vi "P4CMD Compare Files.vi"(4 "version":string, 6 "compare options":T1, 7 "advanced options":variant, 8 "error in (no error)":errorcluster, 9 "compare method":T2 items=["source control provider default", "contents (silent)", "checksum (silent)", "time (silent)"], 10 "file path":path, 11 "source control reference in":T3) -> (0 "error out":errorcluster, 2 "status message":string, 3 "source control reference out":T3, 5 "file differs?":bool)   [LabVIEW 2020, in "NI_SCC_P4CMD.lvlib"]
uses:
  <vilib>/SourceControl/Providers/P4CMD/NI_SCC_P4CMD.lvlib
  <vilib>/SourceControl/sccapi/SCCAPI Refnum.ctl
  <vilib>/SourceControl/sccapi/SCCAPI Compare Method.ctl
  <vilib>/SourceControl/sccapi/SCCAPI Compare Options.ctl
  <vilib>/SourceControl/Providers/P4CMD/P4CMD Operations.ctl
  <vilib>/SourceControl/support/SCCSup Message Strings GLBL.vi
  <vilib>/SourceControl/sccapi/NI_SCC.lvlib
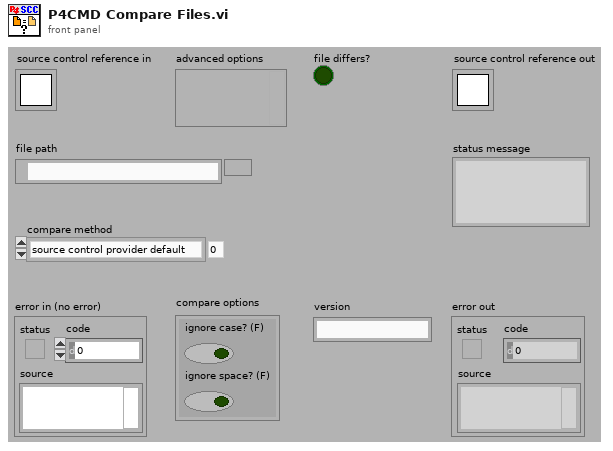
[diagram p1: front panel]
types:
  T1 = typedef "NI_SCC.lvlib/SCCAPI Compare Options.ctl" = cluster{"ignore case? (F)":bool, "ignore space? (F)":bool}
  T2 = typedef "NI_SCC.lvlib/SCCAPI Compare Method.ctl" = u16
  T3 = typedef "NI_SCC.lvlib/SCCAPI Refnum.ctl" = refnum<k1>
  T4 = typedef "NI_SCC_P4CMD.lvlib/P4CMD Operations.ctl" = enum16{"get all clients", "get all users", "describe changelist", "sync from depot", "open for edit", "submit to depot", "revert", "add to depot", "remove from depot", "print files revisions", "compare client file", "print depot file contents", "list opened files", "get file info", "lock files", "edit changelist spec", "info", "set variables"}
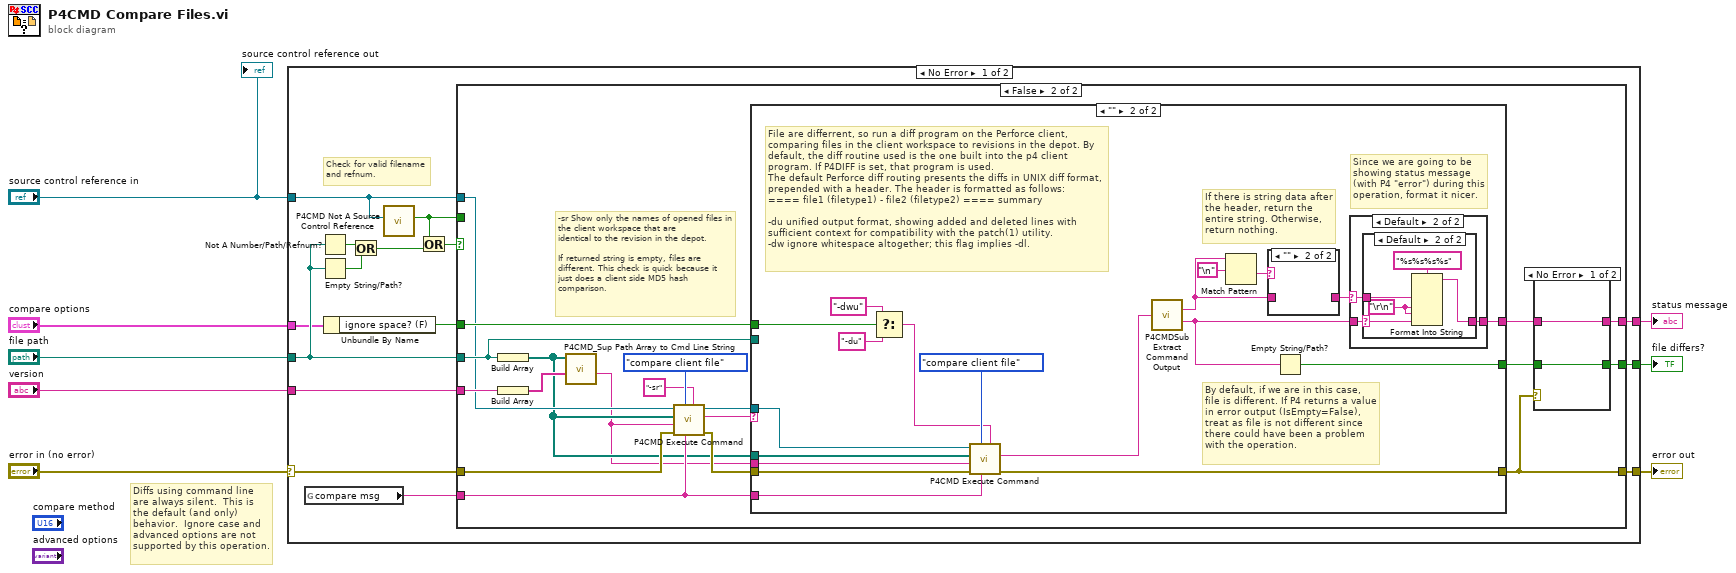
[diagram p0: block diagram]
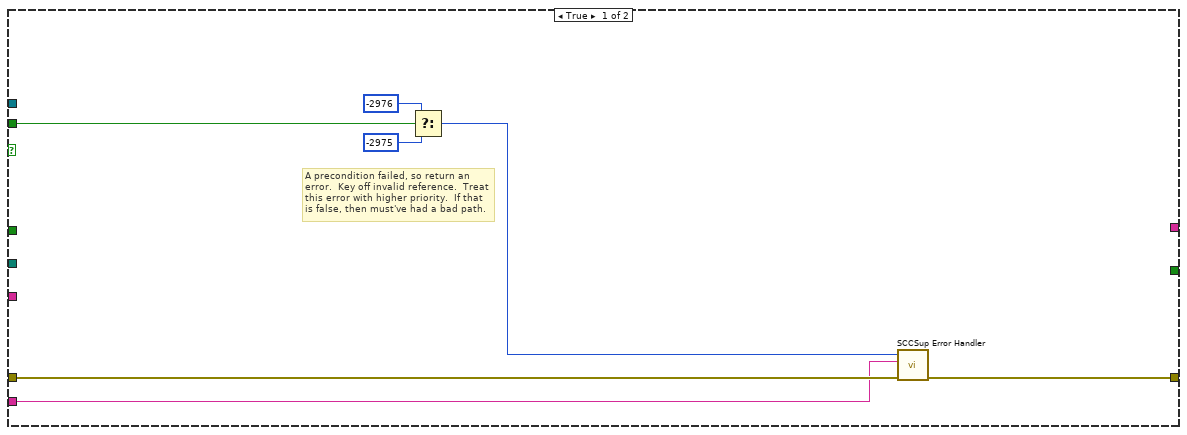
[diagram p2: hidden frame]
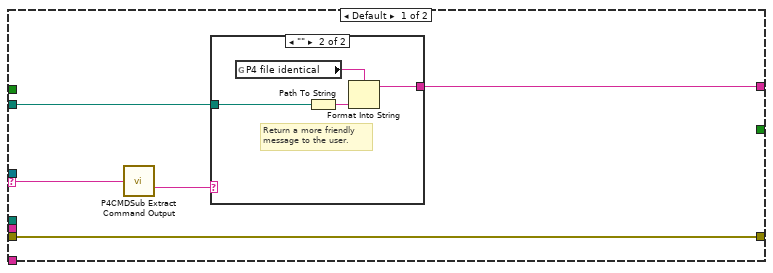
[diagram p4: hidden frame]
diagram:
  # "Diffs using command line are always silent.  This is the default (and only) behavior.  Ignore case and advanced options are not supported by this operation."
  n1 = case shown="No Error" "error in (no error)" {
    selector: "error in (no error)" -> [w15 w92]
    tunnel: [w14 w92] -> w7
    tunnel: "source control reference in" -> [w22 _]
    tunnel: [w23 _] -> w5
    tunnel: "file path" -> [w21 _]
    tunnel: [w12 _] -> w3
    tunnel: "compare options" -> [w11 _]
    tunnel: "version" -> [w9 _]
    frame No Error {
      # "Check for valid filename and refnum."
      n2 = global read "SCCSup Message Strings GLBL.vi" "compare msg"() -> (w13:string)
      n3 = Not A Number/Path/Refnum?(number/path/refnum=w21) -> (NaN/Path/Refnum?=w20:bool)
      n4 = Empty String/Path?(string/path=w21) -> (empty?=w19:bool)
      n5 = Unbundle By Name(w11) -> ("ignore space? (F)"=w10:bool)
      n6 = Or(x=w20, y=w19) -> (x .or. y?=w18:bool)
      n7 = call <vilib>:"P4CMD Not A Source Control Reference.vi"("source control reference in"=w22) -> ("not a source control reference?"=w16:bool)  [unwired: 9 in, 1 out]
      n8 = Or(x=w16, y=w18) -> (x .or. y?=w17:bool)
      n9 = case shown="False" w17 {
        tunnel: w22 -> [_ w40]
        tunnel: [_ w31] -> w23
        tunnel: w21 -> [_ w46]
        tunnel: w10 -> [_ w49]
        tunnel: w16 -> [w30 _]
        tunnel: w15 -> [w27 w43]
        tunnel: [w26 w35] -> w14
        tunnel: w13 -> [w25 w42]
        tunnel: [_ w33] -> w12
        tunnel: w9 -> [_ w48]
        frame True {
          # "A precondition failed, so return an error.  Key off invalid reference.  Treat this error with higher priority.  If that is false, then must've had a bad path."
          n10 = Select(t=-2976 ("result"), s=w30, f=-2975 ("result")) -> (s? t:f=w24:i32)
          n11 = call <vilib>:"SCCSup Error Handler.vi"("error in (no error)"=w27, "operation message"=w25, "scc error code"=w24) -> ("error out"=w26:errorcluster)  [unwired: 8 in]
        }
        frame False {
          # "-sr Show only the names of opened files in the client workspace that are\nidentical to the revision in the depot.\n\nIf returned string is empty, files are different. This check is quick because it just does a client side MD5 hash comparison."
          n12 = Build Array(w46) -> (w38:path[])
          n13 = Build Array(w48) -> (w47:string[])
          n14 = call <vilib>:"P4CMD_Sup Path Array to Cmd Line String.vi"("modifiers"=w47, "files"=w38) -> ("string output"=w37:string)  [unwired: 8 in, 1 out]
          n15 = call <vilib>:"P4CMD Execute Command.vi"("optional operation parameters"="-sr", "operation message"=w42, "p4 operation"=P4CMD_Operations."compare client file", "error in (no error)"=w43, "input string"=w37, "files"=w38, "source control reference in"=w40) -> ("error out"=w41:errorcluster, "command information"=w36:string, "source control reference out"=w39:T3)  [unwired: 2 in]
          n16 = case shown="\"\"" w36 {
            selector: w36 -> [w53 _]
            tunnel: w49 -> [_ w80]
            tunnel: [w56 w79] -> w35
            tunnel: [_ w66] -> w34
            tunnel: [w54 w68] -> w32
            tunnel: w46 -> [w55 _]
            tunnel: w42 -> [_ w73]
            tunnel: w41 -> [w56 w72]
            tunnel: w39 -> [_ w71]
            tunnel: w38 -> [_ w70]
            tunnel: w37 -> [_ w69]
            frame Default {
              n17 = call <vilib>:"P4CMDSub Extract Command Output.vi"("bundled message"=w53) -> ("command error"=w52:string)  [unwired: 13 in, 1 out]
              n18 = case shown="\"\"" w52 {
                selector: w52 -> [w57 _]
                tunnel: w55 -> [_ w59]
                tunnel: [w57 w58] -> w54
                frame Default {
                  # "If message returned in command error, return that info to user. The values range from file not in client view to password not entered, but it's better that this information is shown than return falsely that file is identical."
                }
                frame "" {
                  # "Return a more friendly message to the user."
                  n19 = global read "SCCSup Message Strings GLBL.vi" "P4 file identical"() -> (w60:string)
                  n20 = Path To String(path=w59) -> (string=w61:string)
                  n21 = Format Into String(format string=w60, w61) -> (resulting string=w58:string)  [unwired: 2 in, 1 out]
                }
              }
            }
            frame "" {
              # "If there is string data after the header, return the entire string. Otherwise, return nothing."
              # "Since we are going to be showing status message (with P4 \"error\") during this operation, format it nicer."
              # "By default, if we are in this case, file is different. If P4 returns a value in error output (IsEmpty=False), treat as file is not different since there could have been a problem with the operation."
              # "File are differrent, so run a diff program on the Perforce client, comparing files in the client workspace to revisions in the depot. By default, the diff routine used is the one built into the p4 client program. If P4DIFF is set, that program is used.\nThe default Perforce diff routing presents the diffs in UNIX diff format, prepended with a header. The header is formatted as follows:\n==== file1 (filetype1) - file2 (filetype2) ==== summary\n\n-du unified output format, showing added and deleted lines with sufficient context for compatibility with the patch(1) utility.\n-dw ignore whitespace altogether; this flag implies -dl."
              n22 = Select(t="-dwu", s=w80, f="-du") -> (s? t:f=w74:string)
              n23 = call <vilib>:"P4CMD Execute Command.vi"("optional operation parameters"=w74, "operation message"=w73, "p4 operation"=P4CMD_Operations."compare client file", "error in (no error)"=w72, "input string"=w69, "files"=w70, "source control reference in"=w71) -> ("error out"=w79:errorcluster, "command information"=w78:string)  [unwired: 2 in, 1 out]
              n24 = call <vilib>:"P4CMDSub Extract Command Output.vi"("bundled message"=w78) -> ("command output"=w63:string, "command error"=w67:string)  [unwired: 13 in]
              n25 = Match Pattern(string=w63, regular expression="\n") -> (after substring=w64:string)  [unwired: 1 in, 3 out]
              n26 = case shown="\"\"" w64 {
                tunnel: w63 -> [w81 _]
                tunnel: [w81 _] -> w62
                frame Default {
                }
                frame "" {
                }
              }
              n27 = Empty String/Path?(string/path=w67) -> (empty?=w66:bool)
              n28 = case shown="Default" w62 {
                selector: w62 -> [_ w84]
                tunnel: w67 -> [w82 w83]
                tunnel: [w82 w85] -> w68
                frame "" {
                }
                frame Default {
                  n29 = case shown="Default" w83 {
                    selector: w83 -> [_ w87]
                    tunnel: [w86 w89] -> w85
                    tunnel: w84 -> [w86 w88]
                    frame "" {
                    }
                    frame Default {
                      w90 = "\r\n"
                      n30 = Format Into String(format string="%s%s%s%s", w88, w90, w90, w87) -> (resulting string=w89:string)  [unwired: 2 in, 1 out]
                    }
                  }
                }
              }
            }
          }
          n31 = case shown="No Error" w35 {
            tunnel: [w51 _] -> w33
            tunnel: w34 -> [w51 _]
            tunnel: w32 -> [w50 _]
            tunnel: [w50 _] -> w31
            frame No Error {
            }
            frame Error {
              # "If there was an error, clear outputs."
            }
          }
        }
      }
    }
    frame Error {
    }
  }
  "error out" <- w7
  "status message" <- w5
  "file differs?" <- w3
  "source control reference out" <- "source control reference in"
